vi "GSP_GUI_global.vi"() -> ()   [LabVIEW 2015]
panel:
  in  "Primary Filter Wheel Type":bool caption="Primary FilterWheel"
  in  "User Type":i8
  in  "Standard Observing Mode Names":string[](array[string])
  in  "Standard Observing Modes File":path
  in  "UserFile":path
  in  "Slit File":path
  in  "Filter File":path
  in  "Grating File":path
  in  "Engineering File":path
  in  "Manager Poll Delay":u32=500
  in  "Configuration File":path
  in  "Slit Mask Names":string[](array[string])
  in  "Grating Names":string[](array[string])
  in  "Secondary Filter Names":string[](array[string])
  in  "Primary Filter Names":string[](array[string])
  in  "UserPath":path
  in  "Current User":string
  # "6-hole (ROUND)"
  # "5-hole (SQUARE)"
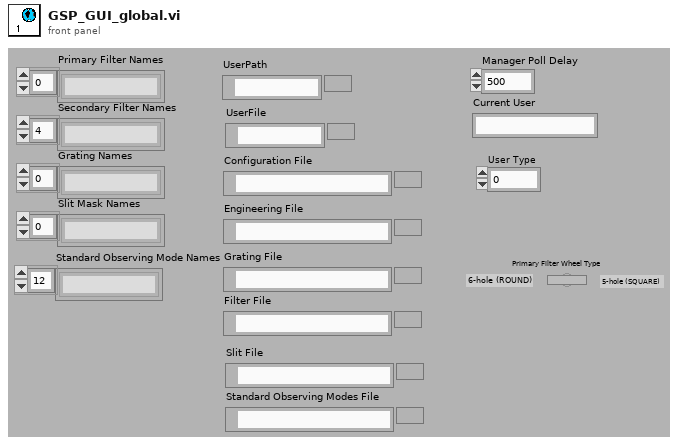
[diagram p1: front panel]
diagram:
